vi "Reposition Multiple Wheels on Steering Frame.vi"(5 "x positions":dbl[](array[numeric]), 6 "frame angles (rad)":dbl[](array[numeric]), 7 "y positions":dbl[](array[numeric]), 8 "error in (no error)":errorcluster, 10 "wheel indexes":i32[](array[numeric]), 11 "steering frame in":refnum<class "NI_Robotics_Steering Frame.lvclass">) -> (0 "error out":errorcluster, 1 "found?":bool[](array[boolean]), 3 "steering frame out":refnum<class "NI_Robotics_Steering Frame.lvclass">)   [LabVIEW 2017, in "NI_Robotics_Steering Frame.lvclass"]
doc: "Changes the location of the wheel or wheels to the position and angle you specify. You must manually select the polymorphic instance to use."
uses:
  <vilib>/robotics/Steering/Steering Frame/NI_Robotics_Steering Frame.lvclass
  <vilib>/robotics/Steering/Steering Frame/NI_Robotics_Steering Frame.lvclass/NI_Robotics_Steering Frame.ctl
  <vilib>/robotics/Steering/Wheel/NI_Robotics_Wheel.lvclass/NI_Robotics_Wheel.ctl
  <vilib>/robotics/Steering/Wheel/Update Steering to Wheel Frame Transform.vi
  <vilib>/Analysis/coordinate.llb/Wrap Angle.vi
  <vilib>/Analysis/coordinate.llb/Wrap Angle (scalar).vi
  <vilib>/robotics/Utilities/NI_Robotics Utilities.lvlib
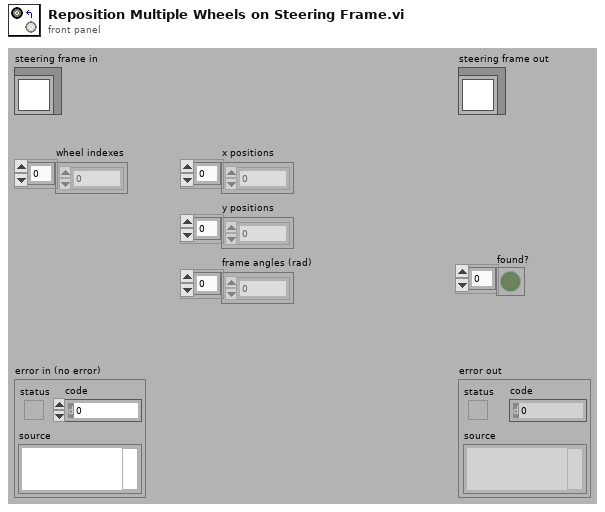
[diagram p1: front panel]
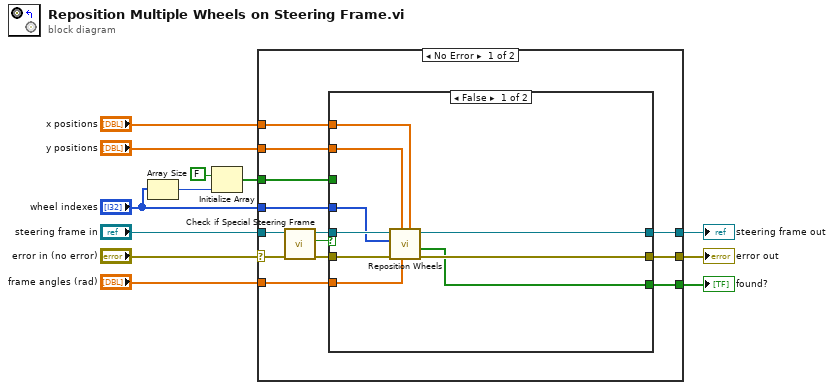
[diagram p0: block diagram]
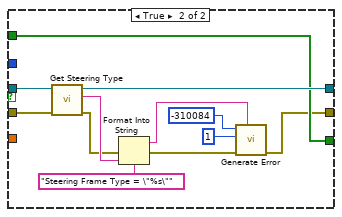
[diagram p2: hidden frame]
diagram:
  n1 = Array Size(array="wheel indexes") -> (size(s)=w1:i32)
  n2 = Initialize Array(FALSE, w1) -> (w6:bool[])
  n3 = case shown="No Error" "error in (no error)" {
    selector: "error in (no error)" -> [w24 w49]
    tunnel: [w19 w49] -> w11
    tunnel: [w20 w48] -> w9
    tunnel: "steering frame in" -> [w25 w48]
    tunnel: "wheel indexes" -> [w18 _]
    tunnel: w6 -> [w17 w47]
    tunnel: [w16 w47] -> w5
    tunnel: "x positions" -> [w15 _]
    tunnel: "y positions" -> [w14 _]
    tunnel: "frame angles (rad)" -> [w13 _]
    frame No Error {
      n4 = call-dynamic "Check if Special Steering Frame.vi"("error in (no error)"=w24, "steering frame in"=w25) -> ("error out"=w21:errorcluster, "special?"=w23:bool, "steering frame out"=w22:refnum<class "NI_Robotics_Steering Frame.lvclass">)  [unwired: 7 in]
      n5 = case shown="False" w23 {
        tunnel: w22 -> [w34 w39]
        tunnel: w21 -> [w33 w38]
        tunnel: [w28 w37] -> w20
        tunnel: [w27 w35] -> w19
        tunnel: w18 -> [w32 _]
        tunnel: w17 -> [_ w36]
        tunnel: [w26 w36] -> w16
        tunnel: w15 -> [w30 _]
        tunnel: w14 -> [w31 _]
        tunnel: w13 -> [w29 _]
        frame False {
          n6 = call <vilib>:"Reposition Wheels.vi"("x positions"=w30, "frame angles (rad)"=w29, "y positions"=w31, "error in (no error)"=w33, "wheel indexes"=w32, "steering frame in"=w34) -> ("error out"=w27:errorcluster, "found?"=w26:bool[], "steering frame out"=w28:refnum<class "NI_Robotics_Steering Frame.lvclass">)  [unwired: 3 in]
        }
        frame True {
          n7 = call-dynamic "Get Steering Type.vi"("error in (no error)"=w38, "steering frame in"=w39) -> ("error out"=w42:errorcluster, "steering type"=w44:string, "steering frame out"=w37:refnum<class "NI_Robotics_Steering Frame.lvclass">)  [unwired: 7 in]
          n8 = Format Into String(format string="Steering Frame Type = \"%s\"", error in=w42, w44) -> (resulting string=w45:string, error out=w43:errorcluster)  [unwired: 1 in]
          n9 = call <vilib>:"Generate Error.vi"("<append> (\"\")"=w45, "error in (no error)"=w43, "chain levels to remove (1)"=1, "code"=-310084) -> ("error out"=w35:errorcluster)  [unwired: 7 in]
        }
      }
    }
    frame Error {
    }
  }
  "error out" <- w11
  "steering frame out" <- w9
  "found?" <- w5
